vi "Reinitialize.vi"(8 "error in (no error)":errorcluster, 11 "MKS MW in":refnum<class "PL MKS MW.lvclass">) -> (0 "error out":errorcluster, 3 "MKS MW out":refnum<class "PL MKS MW.lvclass">)   [LabVIEW 2015, in "PL MKS MW.lvclass"]
doc: "Reinitializes connection to device based on previously specified settings."
uses:
  PL MKS MW.lvclass
  PL MKS MW.lvclass/PL MKS MW.ctl
  <vilib>/Instr/_visa.llb/VISA Configure Serial Port (Instr).vi
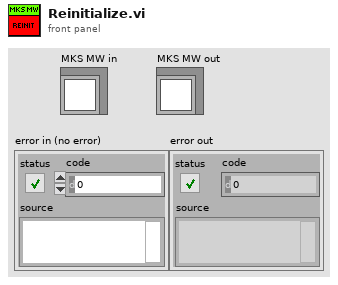
[diagram p1: front panel]
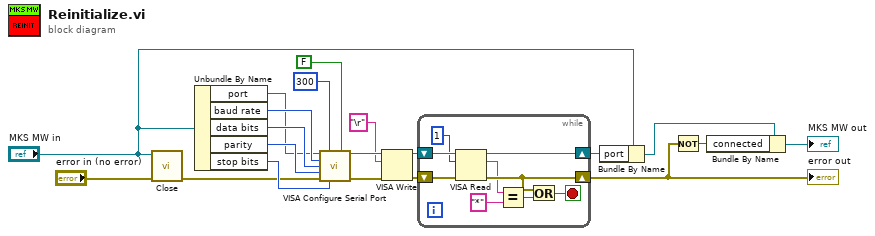
[diagram p0: block diagram]
diagram:
  n1 = call "Close.vi"("error in (no error)"="error in (no error)", "Comdel in"="MKS MW in") -> ("error out"=w9:errorcluster)  [unwired: 9 in]
  n2 = Unbundle By Name("MKS MW in") -> ("port"=w10:refnum<visa-resource-name>, "baud rate"=w15:u32, "data bits"=w14:u16, "parity"=w13:u16, "stop bits"=w12:u16)
  n3 = call-poly "VISA Configure Serial Port"("VISA resource name"=w10, "timeout (10sec)"=u32 300, "Enable Termination\nChar (T)"=FALSE ("Enable Termination\nChar (T)"), "baud rate (9600)"=w15, "data bits (8)"=w14, "parity (0:none)"=w13, "error in (no error)"=w9, "stop bits (10: 1 bit)"=w12) -> ("VISA resource name out"=w8:refnum<visa-resource-name>, "error out"=w7:errorcluster)  [unwired: 6 in]
  n4 = VISA Write(VISA resource name=w8, write buffer="\r", error in (no error)=w7) -> (VISA resource name out=w6:refnum<visa-resource-name>, error out=w4:errorcluster)  [unwired: 1 out]
  n5 = while {
    shift-right: [w27] -> w3
    shift-left: w6 -> [w29]
    shift-right: [w25] -> w2
    shift-left: w4 -> [w28]
    stop <- w24 stop-if-true
    n6 = VISA Read(VISA resource name=w29, byte count=u32 1, error in (no error)=w28) -> (VISA resource name out=w27:refnum<visa-resource-name>, read buffer=w22:string, error out=w25:errorcluster)  [unwired: 1 out]
    n7 = Equal?(x=w22, y="*") -> (x = y?=w23:bool)
    n8 = Or(x=w25, y=w23) -> (x .or. y?=w24:bool)
  }
  "error out" <- w2
  n9 = Bundle By Name(cluster="MKS MW in", "port"=w3) -> (w19:refnum<class "PL MKS MW.lvclass">)
  n10 = Not(x=w2) -> (.not. x?=w18:bool)
  n11 = Bundle By Name(cluster=w19, "connected"=w18) -> (→"MKS MW out":refnum<class "PL MKS MW.lvclass">)
